vi "ReceiverTCp.vi"() -> ()   [LabVIEW 2023]
panel:
  out "data out":string
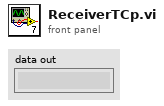
[diagram p1: front panel]
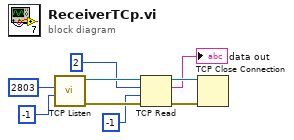
[diagram p0: block diagram]
diagram:
  n1 = call <vilib>:"TCP Listen.vi"("timeout ms (wait forever: -1)"=-1 ("timeout ms (60000)"), "port"=u16 2803 ("remote port or service name")) -> ("error out"=w6:errorcluster, "connection ID"=w7:refnum<k5>)  [unwired: 5 in, 3 out]
  n2 = TCP Read(connection ID=w7, bytes to read=2, error in (no error)=w6, 9:-1 ("timeout ms (25000)")) -> (connection ID out=w9:refnum<k5>, data out=→"data out":string, error out=w8:errorcluster)  [unwired: 1 in]
  n3 = TCP Close Connection(connection ID=w9, error in (no error)=w8) -> ()  [unwired: 1 in, 2 out]
